vi "Read D-Register.vi"(8 "error in":errorcluster, 10 "D-register number":u32=1, 11 "VISA resource name":refnum<visa-resource-name>) -> (0 "error out":errorcluster, 2 "Data":i16, 3 "VISA resource name out":refnum<visa-resource-name>, 4 "Responce (original)":string, 5 "Data Valid":bool)   [LabVIEW 2015, in "Samwontech TEMP2xxx.lvlib"]
uses:
  Samwontech TEMP2xxx.lvlib
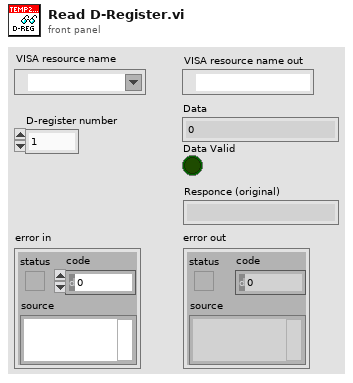
[diagram p1: front panel]
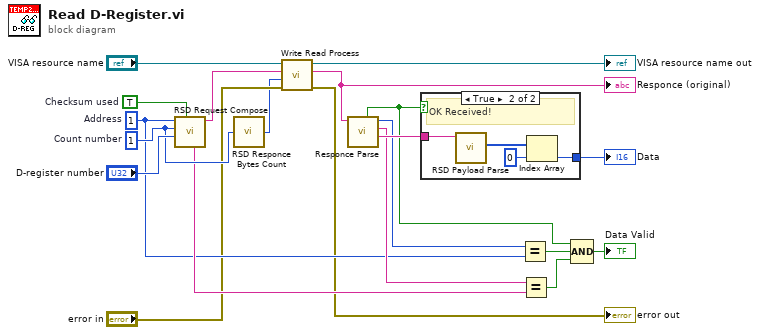
[diagram p0: block diagram]
diagram:
  w18 = u8 1  # Count number
  w12 = u8 1  # Address
  w20 = TRUE  # Checksum used
  n1 = call "RSD Request Compose.vi"("Checksum used"=w20, "D-register number"="D-register number", "Count number"=w18, "Address"=w12) -> ("Request"=w2:string, "Command"=w14:string)  [unwired: 6 in]
  n2 = call "RSD Responce Bytes Count.vi"("Count Number"=w18) -> ("Bytes Count"=w3:u32)
  n3 = call "Write Read Process.vi"("error in (no error)"="error in", "Responce Bytes Count Required"=w3, "Request"=w2, "VISA Refnum in"="VISA resource name") -> ("error out"=→"error out":errorcluster, "Responce"=w5:string, "VISA Refnum out"=→"VISA resource name out":refnum<visa-resource-name>)  [unwired: 4 in, 1 out]
  "Responce (original)" <- w5
  n4 = call "Responce Parse.vi"("Responce"=w5) -> ("Payload"=w16:string, "Command"=w15:string, "Address"=w13:u8, "OK"=w9:bool)  [unwired: 4 in, 3 out]
  n5 = case shown="True" w9 {
    tunnel: [_ w21] -> w17
    tunnel: w16 -> [_ w22]
    frame False {
    }
    frame True {
      # "OK Received!"
      n6 = call "RSD Payload Parse.vi"("Payload"=w22) -> ("Data (number)"=w24:i16[])  [unwired: 9 in, 1 out]
      n7 = Index Array(array=w24, index=0) -> (element=w21:i16)
    }
  }
  "Data" <- w17
  n8 = Equal?(x=w13, y=w12) -> (x = y?=w10:bool)
  n9 = Equal?(x=w15, y=w14) -> (x = y?=w11:bool)
  n10 = Compound Arithmetic op=AND(w9, w10, w11) -> (→"Data Valid":bool)
